vi "niRFUtil CONV 1 Ohm Voltage to dBm (complex array).vi"(2 "Reduced Precision?":bool, 7 "Complex Array (V)":T2 format="%.2f") -> (8 "Real Array (dBm)":T1 min=0 max=127 format="%.2f")   [LabVIEW 2015, in "niRFUtil.lvlib"]
doc: "(c) Copyright 2006, National Instruments, Inc. This VI may not be duplicated, sold, or distributed without written consent from National Instruments."
uses:
  niRFUtil.lvlib
  Includes/niRFUtil INC Complex Array.ctl
  Includes/niRFUtil INC Real Array.ctl
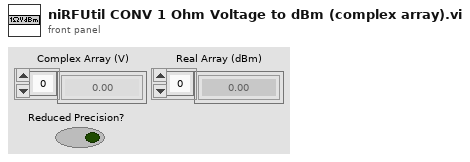
[diagram p1: front panel]
types:
  T1 = typedef "niRFUtil.lvlib/niRFUtil INC Real Array.ctl" = sgl[]
  T2 = typedef "niRFUtil.lvlib/niRFUtil INC Complex Array.ctl" = csg[]
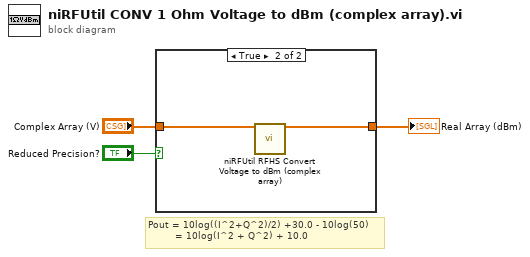
[diagram p0: block diagram]
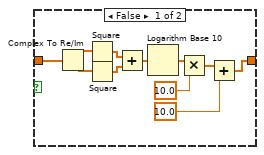
[diagram p2: hidden frame]
diagram:
  # "Pout = 10log((I^2+Q^2)/2) +30.0 - 10log(50)\n         = 10log(I^2 + Q^2) + 10.0"
  n1 = case shown="True" "Reduced Precision?" {
    tunnel: [w4 w15] -> w2
    tunnel: "Complex Array (V)" -> [w5 w16]
    frame False {
      n2 = Complex To Re/Im(x + iy=w5) -> (x=w10:sgl[], y=w9:sgl[])
      n3 = Square(x=w10) -> (x^2=w8:sgl[])
      n4 = Square(x=w9) -> (x^2=w7:sgl[])
      n5 = Add(x=w8, y=w7) -> (x+y=w6:sgl[])
      n6 = Logarithm Base 10(1:w6) -> (0:w14:sgl[])
      n7 = Multiply(x=w14, y=sgl 10.0) -> (x*y=w12:sgl[])
      n8 = Add(x=w12, y=sgl 10.0) -> (x+y=w4:sgl[])
    }
    frame True {
      n9 = call "niRFUtil RFHS Convert Voltage to dBm (complex array).vi"("Complex Array (V)"=w16) -> ("Real Array (dBm)"=w15:T1)  [unwired: 14 in]
    }
  }
  "Real Array (dBm)" <- w2
